vi "UI.vi"(9 "Steps":string[][](array[string]), 10 "Sequences":string[](array[string])) -> ()   [LabVIEW 2015, in "Sequencer Module tests.lvlib"]
uses:
  Sequencer Module tests.lvlib
  module/execution/Sequencer State Enum.ctl
  classes/Step/Execution/Step Status.ctl
  classes/Step/Execution/Step Flow Control.ctl
  module/execution/Sequencer Module runtime.lvclass
  classes/Step/Execution/Step.lvclass
panel:
  out "Sequencer State I32":i32=2
  out "Steps":i32(listbox)
  out "Sequences":i32(listbox)
  out "Active Step UI Alias":string
  out "Active Step":i32
  out "Done":bool
  out "Jump Index":i32
  out "Flow Control":T1
  out "Step State":T2
  out "Sequence #":i32
  out "Active Sequence Name":string
  out "Sequencer State":T3=enum."Start Sequence"
  out "ctl Done":bool
  out "i":i32
  out "LED 2":bool
  out "LED 1":bool
  in  "Boolean 1":bool
  in  "Boolean 0":bool
  in  "Serial Number":string
  in  "Terminate":bool
  in  "Abort":bool
  in  "Pause":bool
  in  "New Sequence":i32
  in  "Change Sequence":bool
  in  "Start":bool
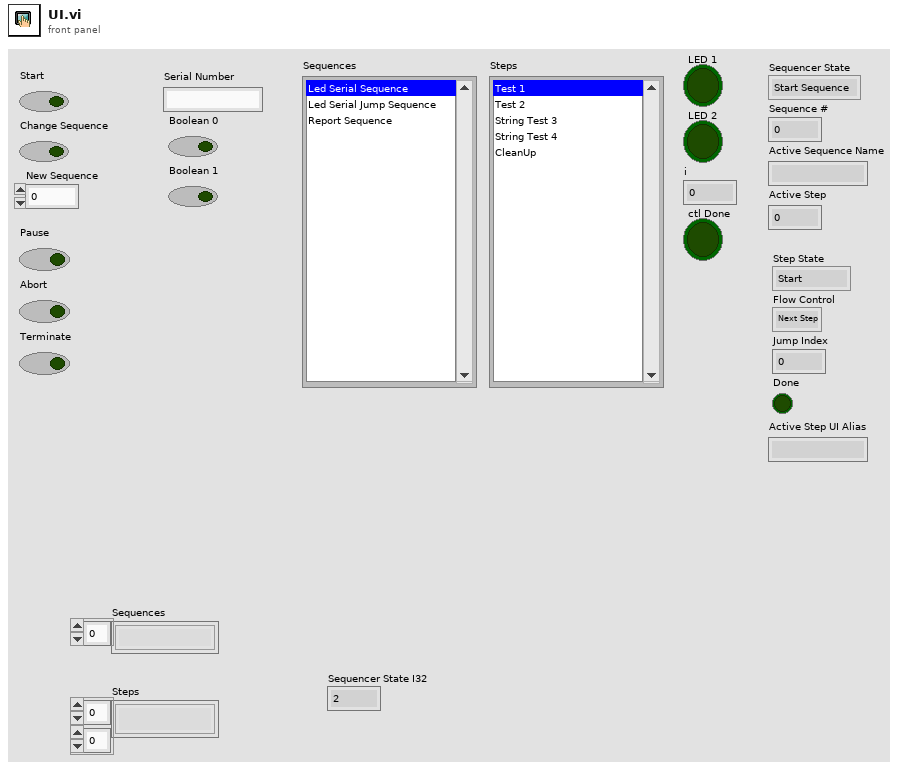
[diagram p1: front panel]
types:
  T1 = typedef "Step.lvclass/Step Flow Control.ctl" = enum16{"Next Step", "Jump"}
  T2 = typedef "Step.lvclass/Step Status.ctl" = enum16{"Start", "Passed", "Failed", "Error", "Done", "Terminated", "Skipped", "Running"}
  T3 = typedef "Sequencer Module runtime.lvclass/Sequencer State Enum.ctl" = enum16{"Idle", "Paused", "Start Sequence", "Run Sequence", "CleanUp Sequence", "Generate Report"}
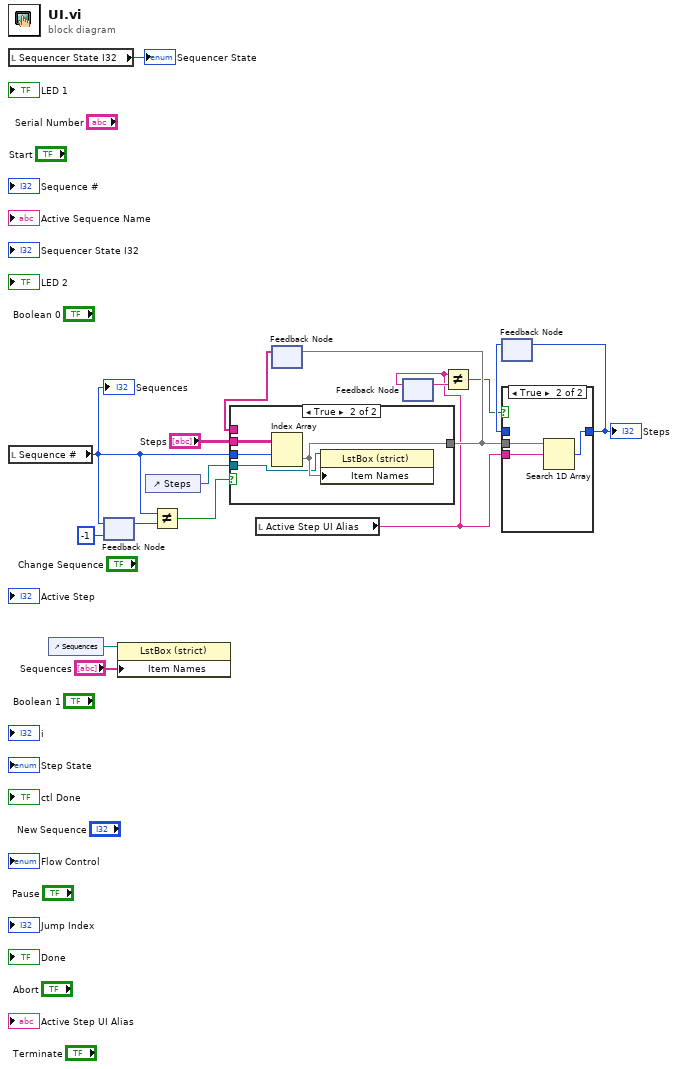
[diagram p0: block diagram]
diagram:
  n1 = local read "Sequencer State I32"() -> (→"Sequencer State":i32)
  n2 = local read "Sequence #"() -> (w8:i32)
  "Sequences" <- w8
  n3 = control-ref of="Sequences"() -> (w3:refnum<vi>)
  n4 = feedback #1(-1 ("Sequence #")) -> (w10:i32)
  n5 = feedback-in #1(w8) -> ()
  n6 = property on="Property Node" class="LstBox (strict)"(reference=w3, "Item Names"="Sequences") -> ()  [unwired: 1 in, 2 out]
  n7 = control-ref of="Steps"() -> (w6:refnum<vi>)
  n8 = Not Equal?(x=w8, y=w10) -> (x != y?=w11:bool)
  n9 = local read "Active Step UI Alias"() -> (w9:string)
  n10 = feedback #2() -> (w12:string[])  [unwired: 1 in]
  n11 = case shown="True" w11 {
    tunnel: "Steps" -> [_ w21]
    tunnel: w8 -> [_ w20]
    tunnel: [w17 w19] -> w15
    tunnel: w12 -> [w17 _]
    tunnel: w6 -> [_ w18]
    frame False {
    }
    frame True {
      n12 = Index Array(array=w21, index (row)=w20) -> (element=w19:string[])  [unwired: 1 in]
      n13 = property on="Property Node" class="LstBox (strict)"(reference=w18, "Item Names"=w19) -> ()  [unwired: 1 in, 2 out]
    }
  }
  n14 = feedback-in #2(w15) -> ()
  n15 = feedback #3() -> (w13:string)  [unwired: 1 in]
  n16 = feedback-in #3(w9) -> ()
  n17 = Not Equal?(x=w9, y=w13) -> (x != y?=w14:bool)
  n18 = feedback #4() -> (w16:i32)  [unwired: 1 in]
  n19 = case shown="True" w14 {
    tunnel: w15 -> [_ w25]
    tunnel: w9 -> [_ w24]
    tunnel: [w22 w23] -> w5
    tunnel: w16 -> [w22 _]
    frame False {
    }
    frame True {
      n20 = Search 1D Array(1D array=w25, element=w24) -> (index of element=w23:i32)  [unwired: 1 in]
    }
  }
  "Steps" <- w5
  n21 = feedback-in #4(w5) -> ()
